vi "PH_Tektronix_7000.set Acquisition GUI Element.vi"(2 "Ref Acqu Config":refnum<vi>, 3 "Acqu Config":T1={"Record Length"=10000, "Timebase [s/div]"=4.0, "Position [%]"=0.0, "Acquisition Type"=0, "Average Waveforms"=10, "Envelope Waveforms"=10, "WfmDB Samples"=16000, "Continuous?"=FALSE, "Delay [s]"=0.0, "Run?"=FALSE} {"Delay [s]" format="%#_12p"; "Acquisition Type" items=["Sample", "Peak Detect", "Hi Res", "Average", "Envelope", "WfmDB"]; "Timebase [s/div]" format="%#_12g"}, 4 "enabled?":bool, 5 "error in":errorcluster) -> (19 "error out":errorcluster)   [LabVIEW 2014, in "PH_Tektronix_7000.lvlib"]
doc: "If the reference is valid, the incoming data are set to the GUI."
uses:
  PH_Tektronix_7000.lvlib
  PH_Tektronix_7000.Acquisition Config.ctl
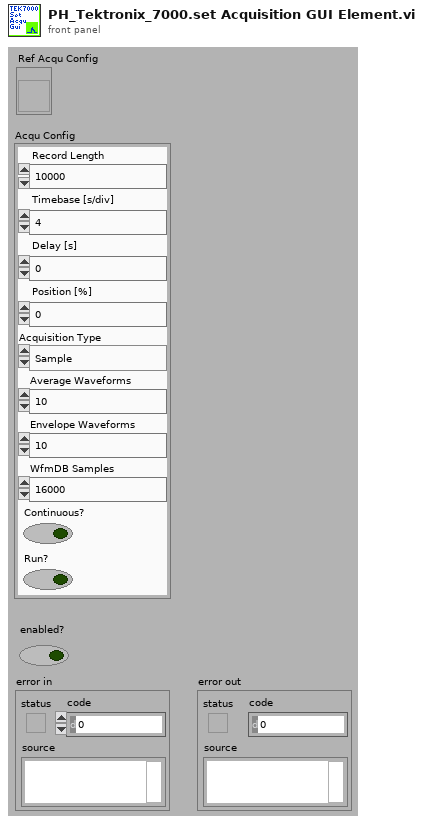
[diagram p1: front panel]
types:
  T1 = typedef "PH_Tektronix_7000.lvlib/PH_Tektronix_7000.Acquisition Config.ctl" = cluster{"Record Length":u32, "Timebase [s/div]":dbl, "Position [%]":dbl, "Acquisition Type":u16, "Average Waveforms":i32, "Envelope Waveforms":i32, "WfmDB Samples":i32, "Continuous?":bool, "Delay [s]":dbl, "Run?":bool}
  T2 = enum8{"Enabled", "Disabled", "Disabled and Grayed Out"}
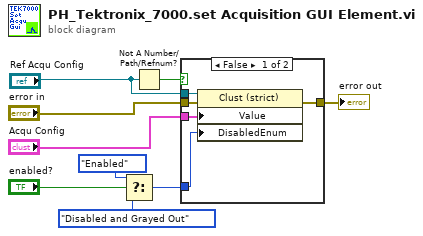
[diagram p0: block diagram]
diagram:
  n1 = Select(t=T2."Enabled" ("Disabled"), s="enabled?", f=T2."Disabled and Grayed Out") -> (s? t:f=w4:T2)
  n2 = Not A Number/Path/Refnum?(number/path/refnum="Ref Acqu Config") -> (NaN/Path/Refnum?=w9:bool)
  n3 = case shown="False" w9 {
    tunnel: "error in" -> [w14 w15]
    tunnel: [w13 w15] -> w7
    tunnel: "Ref Acqu Config" -> [w12 _]
    tunnel: "Acqu Config" -> [w11 _]
    tunnel: w4 -> [w10 _]
    frame False {
      n4 = property class="Clust (strict)"(reference=w12, error in=w14, "Value"=w11, "DisabledEnum"=w10) -> (error out=w13:errorcluster)  [unwired: 1 out]
    }
    frame True {
    }
  }
  "error out" <- w7
